vi "lu_decomposition(SubVI).vi"(10 "Wektor b":dbl[](array[numeric]), 11 "Macierz A":dbl[][](array[numeric])) -> (3 "Wynik":dbl[](array[numeric]))   [LabVIEW 2020]
uses:
  <vilib>/Analysis/BLAS.llb/LV_UpLo.ctl
  <vilib>/addons/Multicore Analysis and Sparse Matrix/Linear Algebra/_linalg/LU Decomposition (DBL).vi
  <vilib>/addons/Multicore Analysis and Sparse Matrix/BLAS/_blas/dgemv - General Matrix-Vector Product (DBL).vi
  <vilib>/Analysis/BLAS.llb/dtrsv - Solve Linear Eqs (Triangle, single) (DBL).vi
  <vilib>/Analysis/NI_AALBLAS.lvlib
  <vilib>/addons/Multicore Analysis and Sparse Matrix/BLAS/NI_MASM_BLAS.lvlib
  <vilib>/addons/Multicore Analysis and Sparse Matrix/Linear Algebra/NI_MASM_MtrxDecomposition.lvlib
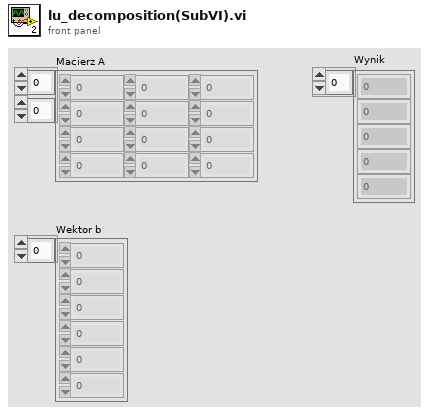
[diagram p1: front panel]
types:
  T1 = typedef "NI_AALBLAS.lvlib/LV_UpLo.ctl" = i32
  T2 = typedef "NI_Matrix.lvlib/RealMatrix.ctl" = dbl[][]
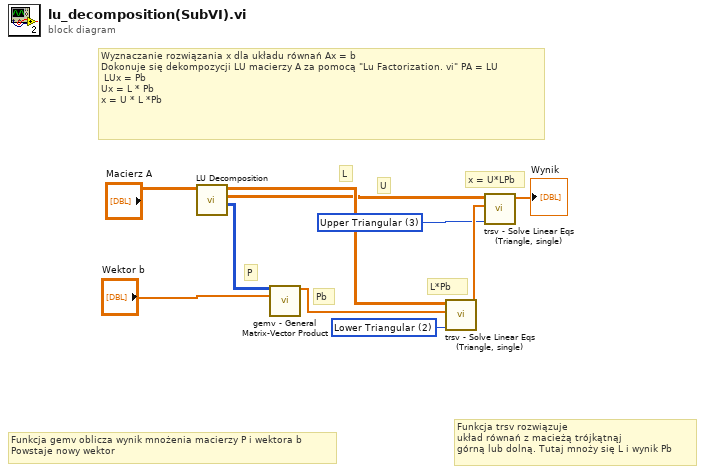
[diagram p0: block diagram]
diagram:
  w2 = T1 2 items=["Lower Triangular"=2, "Upper Triangular"=3] ("matrix A type")
  w3 = T1 3 items=["Lower Triangular"=2, "Upper Triangular"=3] ("matrix A type")
  # "x = U*LPb"
  # "L*Pb"
  # "Pb"
  # "P"
  # "U"
  # "L"
  # "Funkcja gemv oblicza wynik mnożenia macierzy P i wektora b\nPowstaje nowy wektor"
  # "Funkcja trsv rozwiązuje \nukład równań z macieżą trójkątnąj \ngórną lub dolną. Tutaj mnoży się L i wynik Pb"
  # "Wyznaczanie rozwiązania x dla układu równań Ax = b\nDokonuje się dekompozycji LU macierzy A za pomocą \"Lu Factorization. vi\" PA = LU\n LUx = Pb\nUx = L * Pb\nx = U * L *Pb"
  n1 = call-poly <vilib>:"LU Decomposition.vi"("A"="Macierz A") -> ("P"=w8:i32[][], "U"=w6:T2, "L"=w7:T2)  [unwired: 7 in, 1 out]
  n2 = call-poly <vilib>:"gemv - General Matrix-Vector Product.vi"("A"=w8, "x"="Wektor b") -> ("dgemv"=w1:dbl[])  [unwired: 12 in, 1 out]
  n3 = call-poly <vilib>:"trsv - Solve Linear Eqs (Triangle, single).vi"("matrix A type"=w2, "x"=w1, "A"=w7) -> ("dtrsv"=w5:dbl[])  [unwired: 7 in, 1 out]
  n4 = call-poly <vilib>:"trsv - Solve Linear Eqs (Triangle, single).vi"("matrix A type"=w3, "x"=w5, "A"=w6) -> ("dtrsv"=→"Wynik":dbl[])  [unwired: 7 in, 1 out]
